vi "Select Channels Dialog.vi"(7 "Tree header":string="System Channels", 8 "error in (no error)":errorcluster, 9 "Custom Filter":refnum<k24>, 10 "Filter":u8(ring)=1 items=["K_CHAN_R", "K_CHAN_W", "K_CHAN_RW", "K_CHAN_VOLT", "K_CHAN_FAULT", "K_ALL", "K_CUSTOM"], 11 "Start Item Ref":T1=18446744073709551615 format="%.0x") -> (0 "error out":errorcluster, 1 "Canceled":bool, 3 "Channel paths":string[](array[string]))   [LabVIEW 2026, in "Nominal Core Streaming System Explorer.lvlib"]
uses:
  <vilib>/NI VeriStand/Custom Device API/Custom Device Item Ref.ctl
  NationalInstruments.VeriStand.SystemStorage
  Nominal Core Streaming System Explorer.lvlib
  <vilib>/NI VeriStand/Custom Device API/Custom Device API.lvlib
  NationalInstruments.VeriStand.SystemStorageUI
panel:
  in  "OK":bool
  in  "Cancel":bool
  in  "System Channels":refnum<k24>(container)
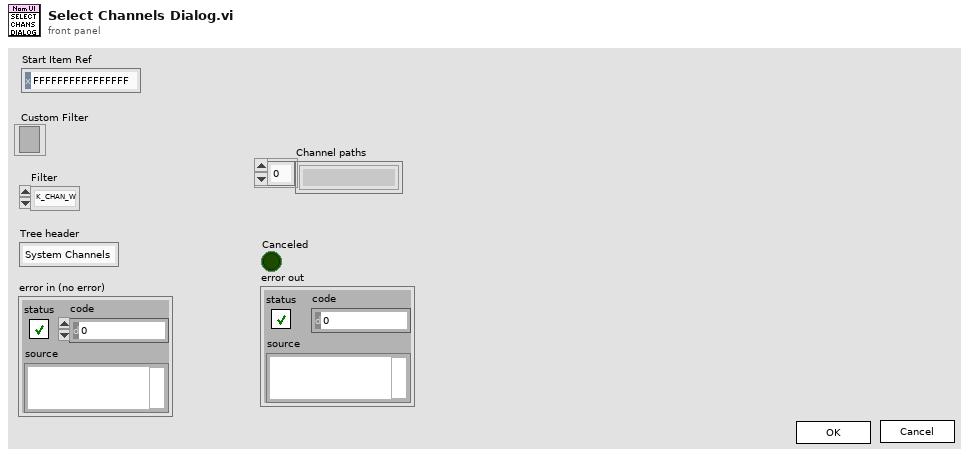
[diagram p1: front panel]
types:
  T1 = typedef "Custom Device API.lvlib/Custom Device Item Ref.ctl" = u64
  T2 = cluster{"Shut Down":bool, "Error":errorcluster, "Root":refnum<k24>, "Cancel":bool, "MapTree":cluster{"Ref":refnum<k24>, "Filter":refnum<k24>}, "Channels":string[]}
  T3 = typedef "Custom Device API.lvlib/Custom Device Pointer.ctl" = refnum<k24>
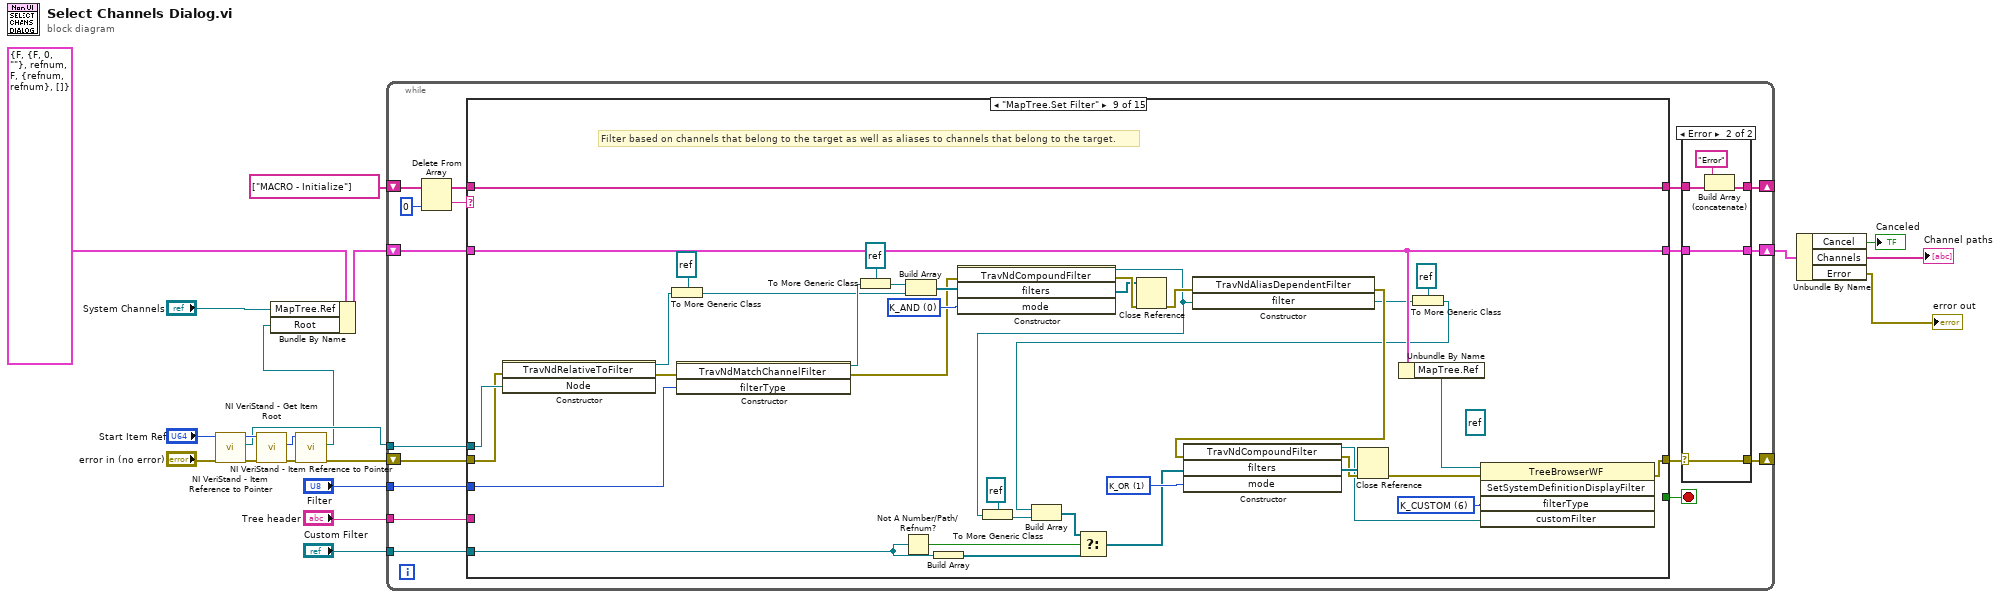
[diagram p0: block diagram]
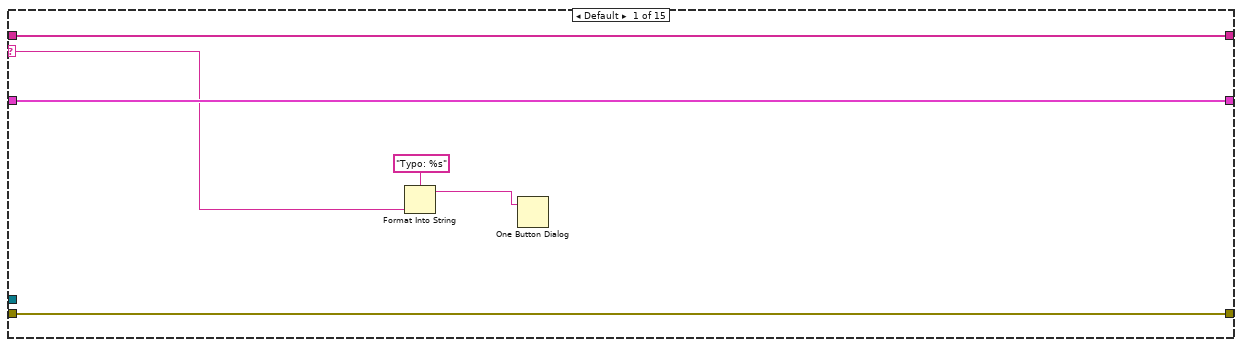
[diagram p3: hidden frame]
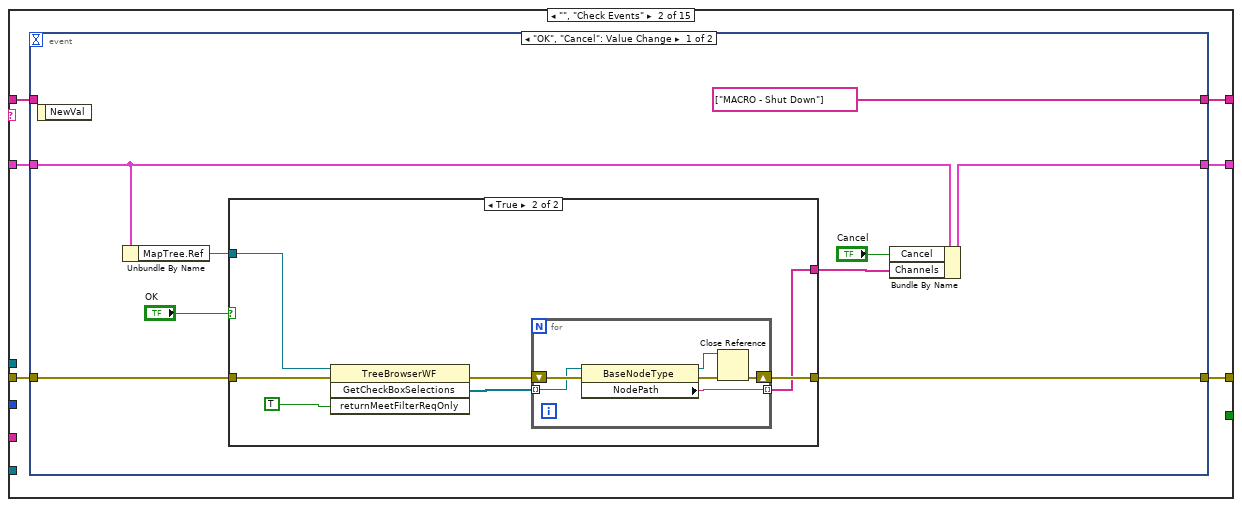
[diagram p4: hidden frame]
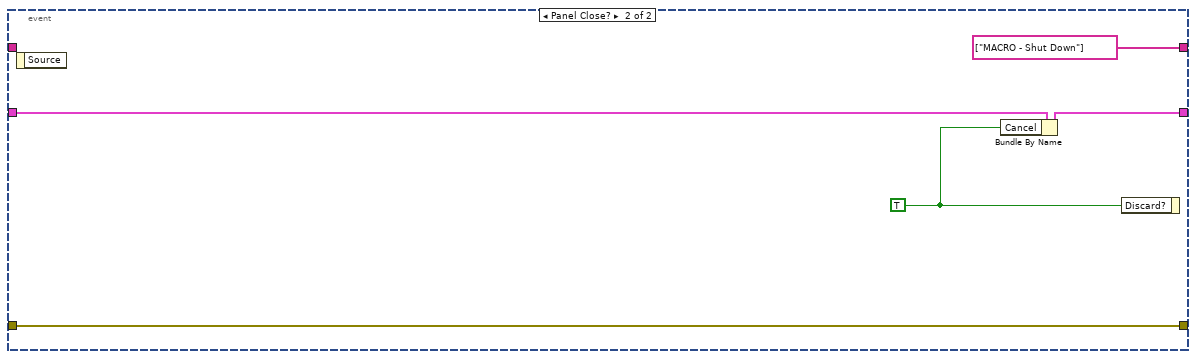
[diagram p6: hidden frame]
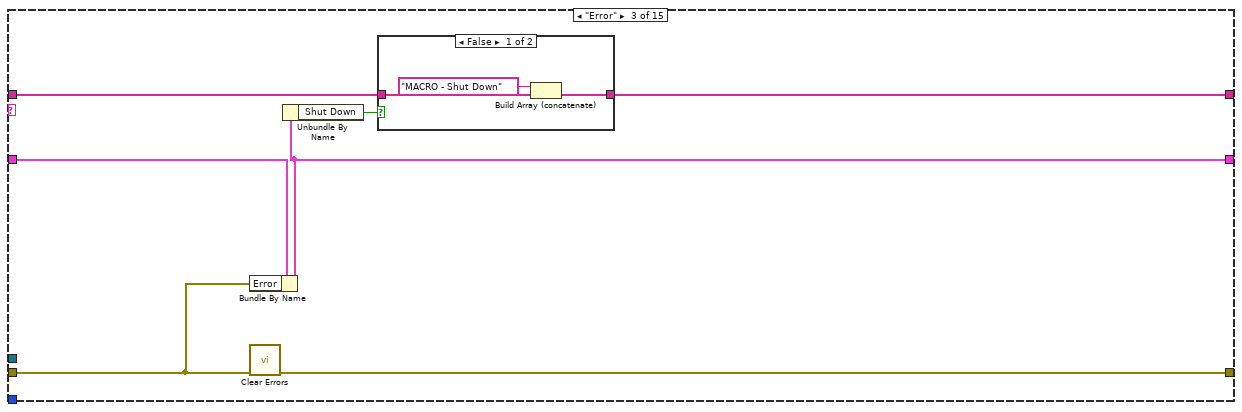
[diagram p7: hidden frame]
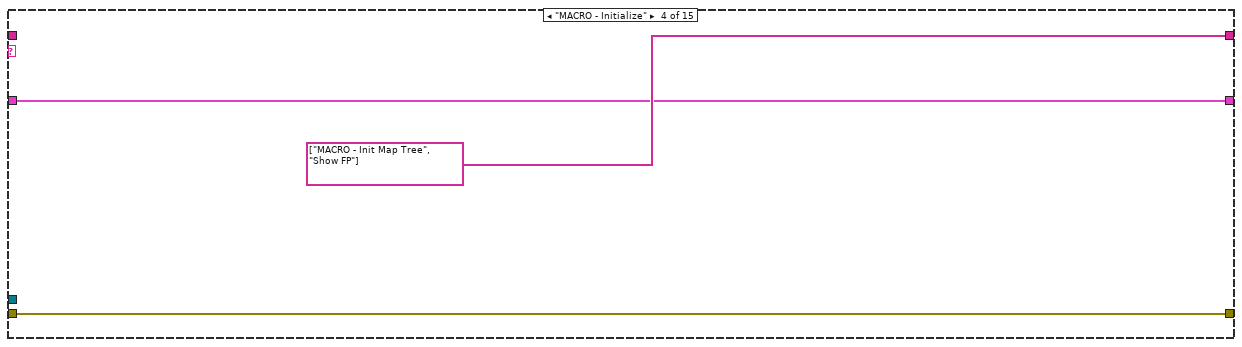
[diagram p9: hidden frame]
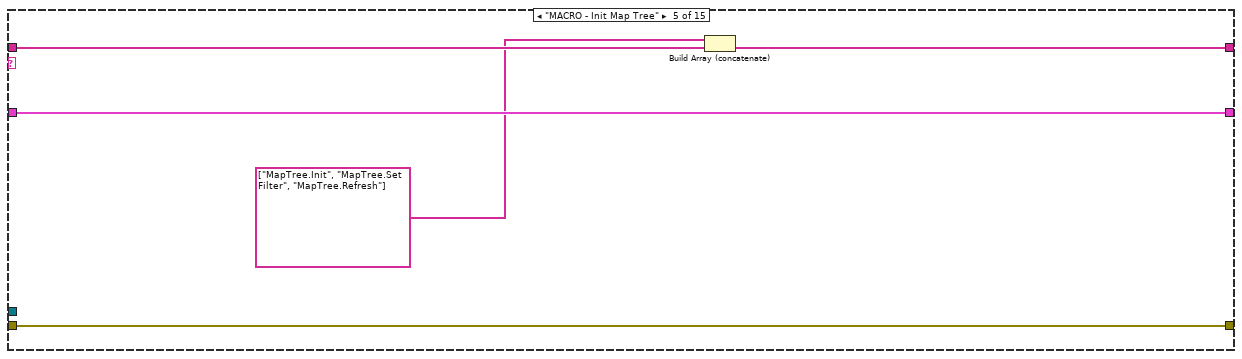
[diagram p10: hidden frame]
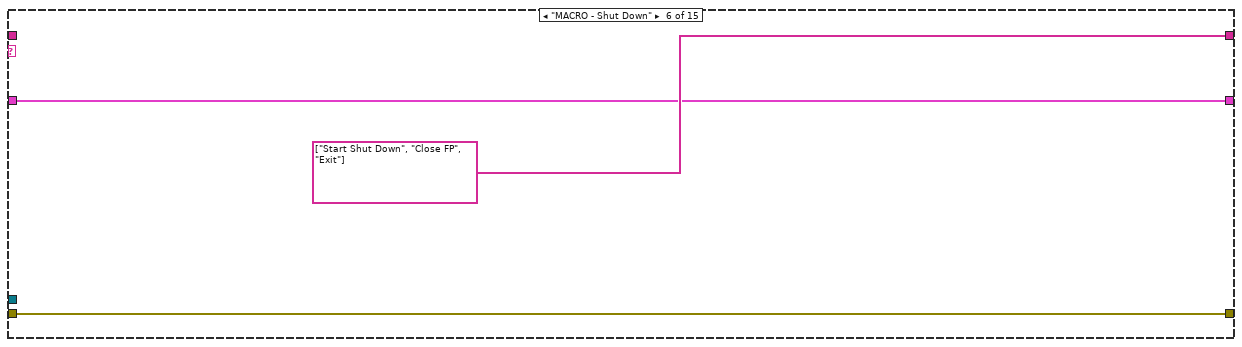
[diagram p11: hidden frame]
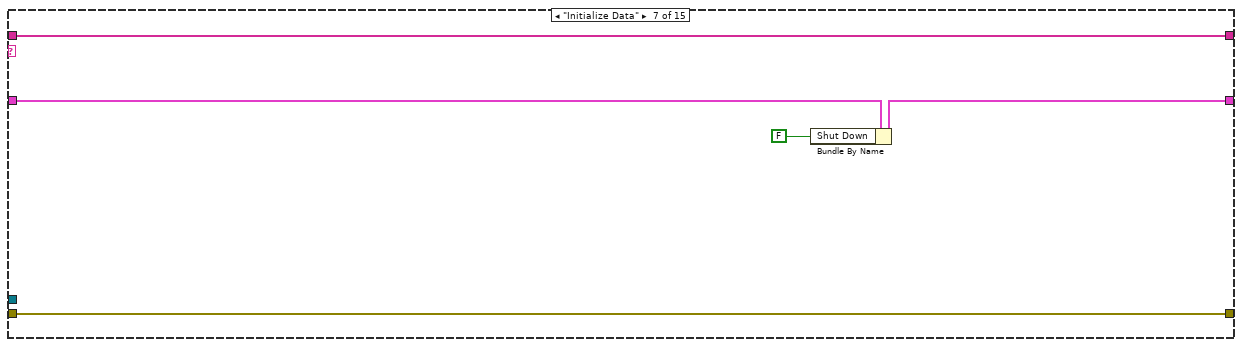
[diagram p12: hidden frame]
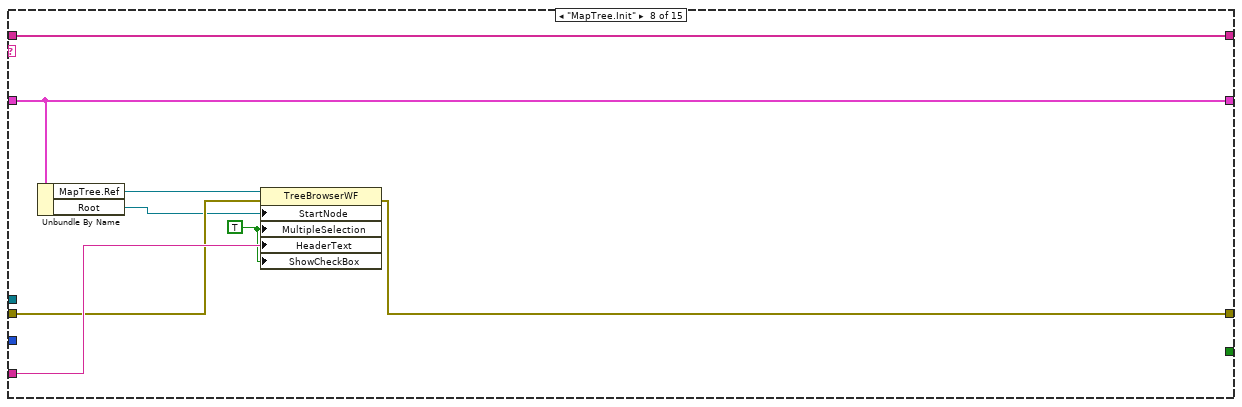
[diagram p13: hidden frame]
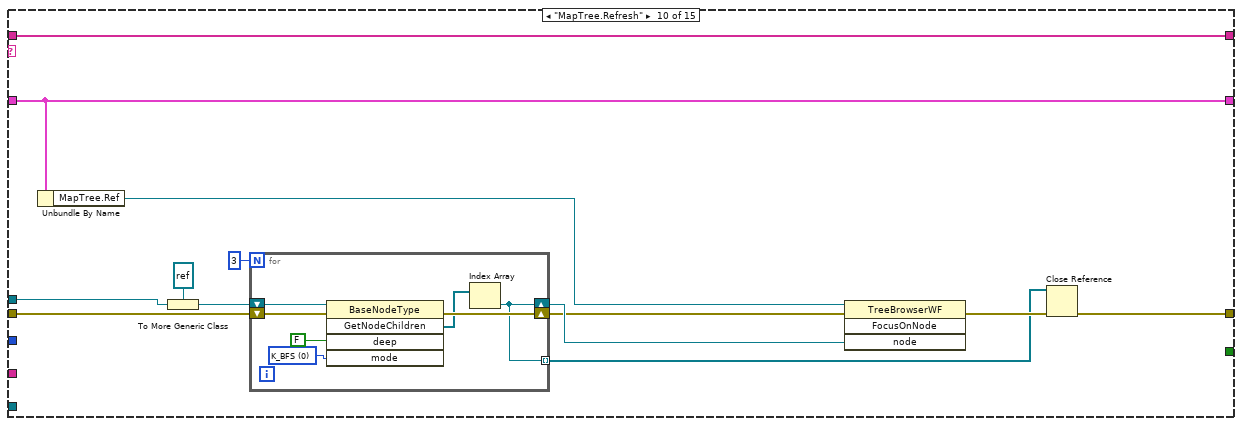
[diagram p14: hidden frame]
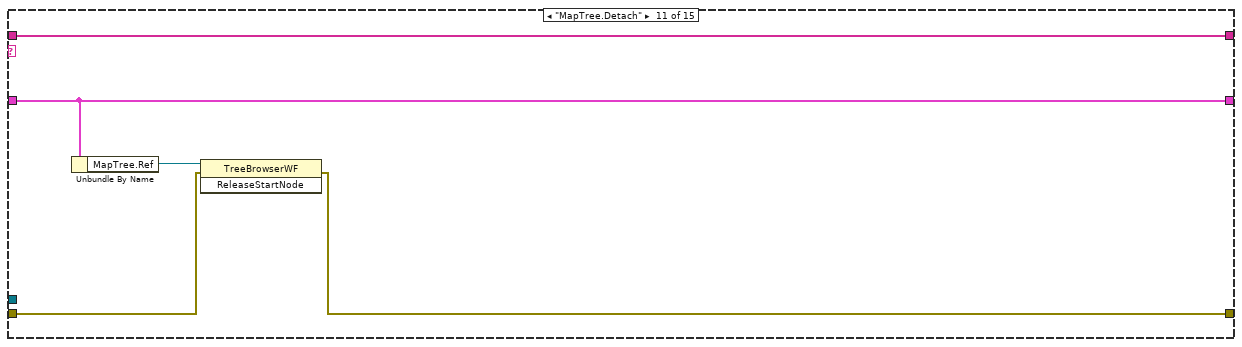
[diagram p15: hidden frame]
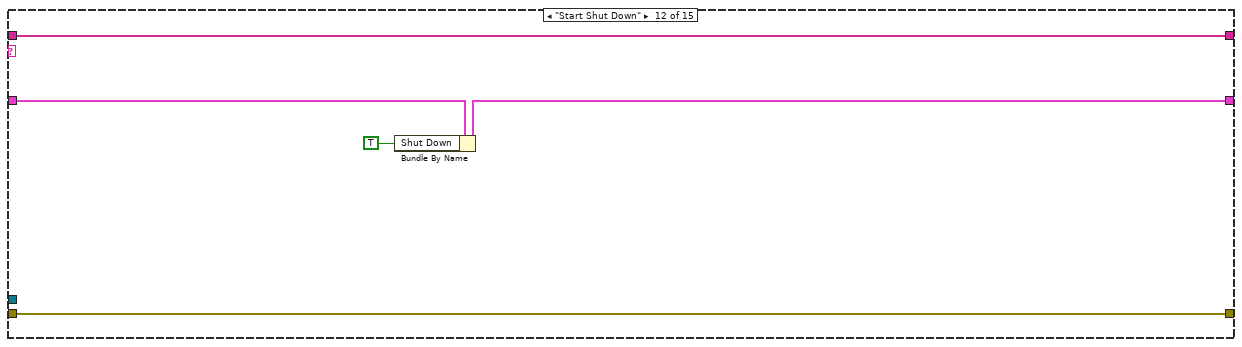
[diagram p16: hidden frame]
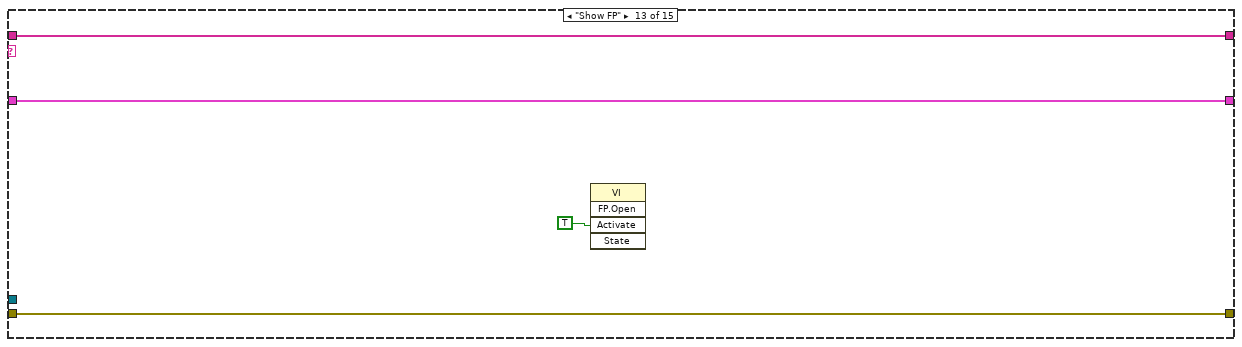
[diagram p17: hidden frame]
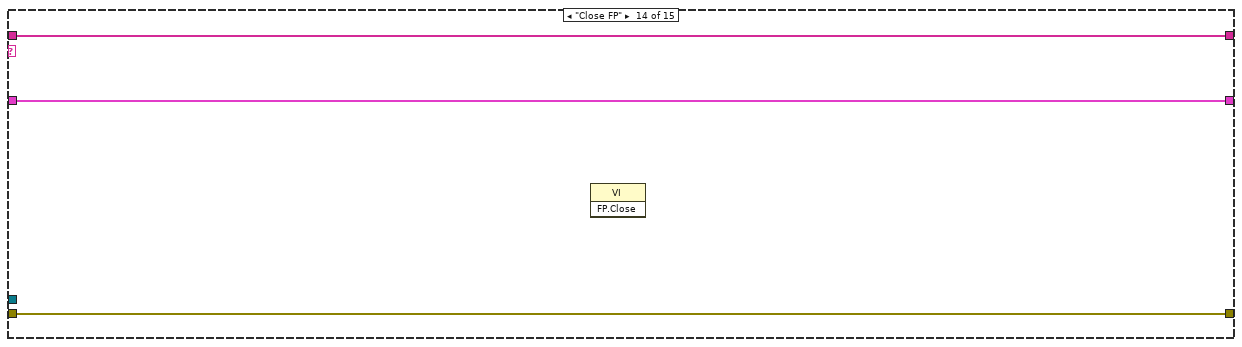
[diagram p18: hidden frame]
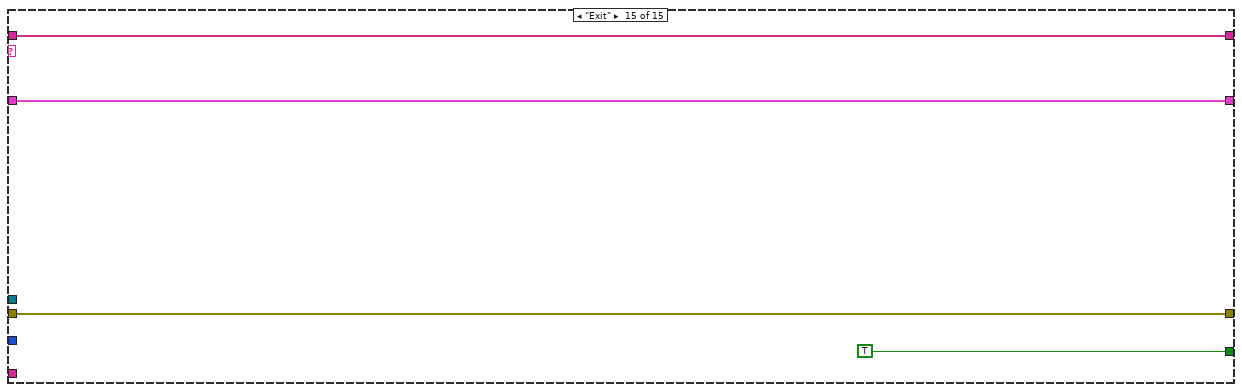
[diagram p19: hidden frame]
diagram:
  n1 = call <vilib>:"NI VeriStand - Item Reference to Pointer.vi"("error in (no error)"="error in (no error)", "Item Ref in"="Start Item Ref") -> ("error out"=w7:errorcluster, "Node Pointer"=w5:T3, "Item Ref out"=w8:T1)  [unwired: 6 in, 1 out]
  n2 = call <vilib>:"NI VeriStand - Get Item Root.vi"("error in (no error)"=w7, "Item Ref in"=w8) -> ("error out"=w4:errorcluster, "Root Ref out"=w1:T1)  [unwired: 6 in, 2 out]
  n3 = call <vilib>:"NI VeriStand - Item Reference to Pointer.vi"("error in (no error)"=w4, "Item Ref in"=w1) -> ("error out"=w3:errorcluster, "Node Pointer"=w2:T3)  [unwired: 6 in, 2 out]
  n4 = Bundle By Name(cluster=T2 {"Shut Down"=FALSE, "Error"={"status"=FALSE, "code"=0, "source"=""}, "Root"=refnum, "Cancel"=FALSE, "MapTree"={"Ref"=refnum, "Filter"=refnum}, "Channels"=[]} ("State Data"), "MapTree.Ref"="System Channels", "Root"=w2) -> (w17:T2)
  n5 = while {
    shift-right: [w27] -> _
    shift-left: string[] ["MACRO - Initialize"] -> [w37]
    shift-right: [w29] -> _
    shift-left: w3 -> [w33]
    shift-right: [w26] -> w13
    shift-left: w17 -> [w31]
    tunnel: "Tree header" -> [w24]
    tunnel: "Filter" -> [w23]
    tunnel: "Custom Filter" -> [w22]
    tunnel: w5 -> [w21]
    stop <- w32 stop-if-true
    n6 = Delete From Array(array=w37, index=0) -> (deleted portion=w34:string, array with subset deleted=w35:string[])  [unwired: 1 in]
    n7 = case shown="\"MapTree.Set Filter\"" w34 {
      selector: w34 -> [w47 _ _ _ _ _ _ _ _ _ _ _ _ _ _]
      tunnel: w35 -> [w51 w57 w89 _ w104 _ w112 w120 w158 w171 w183 w184 w192 w195 w199]
      tunnel: [w51 w52 w88 string[] ["MACRO - Init Map Tree", "Show FP"] ("array") w101 string[] ["Start Shut Down", "Close FP", "Exit"] ("array") w112 w120 w158 w171 w183 w184 w192 w195 w199] -> w28
      tunnel: [w50 w55 w86 w99 w103 w107 w111 w114 w157 w162 w179 w188 w191 w194 w198] -> w30
      tunnel: w33 -> [w50 w54 w87 w99 w103 w107 w111 w115 w129 w169 w180 w188 w191 w194 w198]
      tunnel: [_ _ _ _ _ _ _ _ _ _ _ _ _ _ TRUE] -> w32
      tunnel: w31 -> [w49 w56 w92 w97 w102 w105 w108 w119 w156 w170 w182 w187 w190 w193 w196]
      tunnel: [w49 w53 w91 w97 w102 w105 w110 w119 w156 w170 w182 w186 w190 w193 w196] -> w25
      tunnel: w24 -> [_ _ _ _ _ _ _ w117 _ _ _ _ _ _ _]
      tunnel: w23 -> [_ _ _ _ _ _ _ _ w149 _ _ _ _ _ _]
      tunnel: w22 -> [_ _ _ _ _ _ _ _ w133 _ _ _ _ _ _]
      tunnel: w21 -> [_ _ _ _ _ _ _ _ w145 w159 _ _ _ _ _]
      frame Default {
        n8 = Format Into String(format string="Typo: %s", w47) -> (resulting string=w46:string)  [unwired: 2 in, 1 out]
        n9 = One Button Dialog(message=w46) -> ()  [unwired: 1 in, 1 out]
      }
      frame "", "Check Events" {
        n10 = event shown="[0] \"OK\", \"Cancel\": Value Change" {
          selector: _ -> [_ _]
          dyn-events: _ -> [_ _]
          timeout: _ -> [_ _]
          tunnel: [w59 w85] -> w55
          tunnel: w54 -> [w61 w85]
          tunnel: [w65 w82] -> w53
          tunnel: w56 -> [w63 w84]
          tunnel: w57 -> [_ _]
          tunnel: [string[] ["MACRO - Shut Down"] string[] ["MACRO - Shut Down"]] -> w52
          event "OK", "Cancel": Value Change {
            n11 = event-data() -> ()  [unwired: 1 in, 1 out]
            n12 = Unbundle By Name(w63) -> ("MapTree.Ref"=w62:refnum<k24>)
            n13 = case shown="True" "OK" {
              tunnel: w62 -> [_ w74]
              tunnel: w61 -> [w67 w73]
              tunnel: [_ w68] -> w60
              tunnel: [w67 w69] -> w59
              frame False {
              }
              frame True {
                n14 = invoke class="TreeBrowserWF" method="GetCheckBoxSelections"(reference=w74, error in=w73, "returnMeetFilterReqOnly"=TRUE) -> (error out=w71:errorcluster, "GetCheckBoxSelections"=w70:refnum<k24>[])  [unwired: 1 in, 2 out]
                n15 = for {
                  shift-right: [w75] -> w69
                  shift-left: w71 -> [w80]
                  tunnel: w70 -> [w79] mode=indexing
                  tunnel: [w78] -> w68 mode=indexing
                  n16 = property class="BaseNodeType"(reference=w79, error in=w80) -> (reference out=w76:refnum<k24>, error out=w77:errorcluster, "NodePath"=w78:string)
                  n17 = Close Reference(reference=w76, error in (no error)=w77) -> (error out=w75:errorcluster)
                }
              }
            }
            n18 = Bundle By Name(cluster=w63, "Cancel"="Cancel", "Channels"=w60) -> (w65:T2)
          }
          event Panel Close? {
            w81 = TRUE ("Discard?")
            n19 = event-data() -> ()  [unwired: 1 in, 1 out]
            n20 = Bundle By Name(cluster=w84, "Cancel"=w81) -> (w82:T2)
            n21 = event-data("Discard?"=w81) -> ()  [unwired: 1 in, 1 out]
          }
        }
      }
      frame "Error" {
        n22 = Bundle By Name(cluster=w92, "Error"=w87) -> (w91:T2)
        n23 = call <vilib>:"Clear Errors.vi"("error in (no error)"=w87) -> ("error out"=w86:errorcluster)  [unwired: 5 in, 1 out]
        n24 = Unbundle By Name(w91) -> ("Shut Down"=w90:bool)
        n25 = case shown="False" w90 {
          tunnel: w89 -> [w94 w96]
          tunnel: [w93 w96] -> w88
          frame False {
            n26 = Build Array (concatenate)("MACRO - Shut Down", w94) -> (w93:string[])
          }
          frame True {
            # "Do not interrupt a shut down sequence. This can cause an infinite loop."
          }
        }
      }
      frame "MACRO - Initialize" {
      }
      frame "MACRO - Init Map Tree" {
        n27 = Build Array (concatenate)(string[] ["MapTree.Init", "MapTree.Set Filter", "MapTree.Refresh"] ("array"), w104) -> (w101:string[])
      }
      frame "MACRO - Shut Down" {
      }
      frame "Initialize Data" {
        n28 = Bundle By Name(cluster=w108, "Shut Down"=FALSE) -> (w110:T2)
      }
      frame "MapTree.Init" {
        w116 = TRUE ("MultipleSelection")
        n29 = Unbundle By Name(w119) -> ("MapTree.Ref"=w118:refnum<k24>, "Root"=w113:refnum<k24>)
        n30 = property class="TreeBrowserWF"(reference=w118, error in=w115, "StartNode"=w113, "MultipleSelection"=w116, "HeaderText"=w117, "ShowCheckBox"=w116) -> (error out=w114:errorcluster)  [unwired: 1 out]
      }
      frame "MapTree.Set Filter" {
        (unwired) refnum<k24> refnum ("MapTree.Ref")
        w146 = 0 items=["K_AND", "K_OR"] ("mode")
        w148 = u8 6 items=["K_CHAN_R", "K_CHAN_W", "K_CHAN_RW", "K_CHAN_VOLT", "K_CHAN_FAULT", "K_ALL", "K_CUSTOM", "K_CHAN_R_VIS", "K_CHAN_W_VIS", "K_CHAN_RW_VIS", "K_CHAN_VOLT_VIS", "K_CHAN_FAULT_VIS", "K_WAVE", "K_WAVE_VIS", "K_WAVE_DBL", "K_WAVE_CDB", "K_WAVE_DBL_VIS", "K_WAVE_CDB_VIS"] ("filterType")
        w153 = 1 items=["K_AND", "K_OR"] ("mode")
        # "Filter based on channels that belong to the target as well as aliases to channels that belong to the target."
        n31 = constructor class="TravNdRelativeToFilter"(error in=w129, "Node"=w145) -> (reference out=w142:refnum<k24>, error out=w128:errorcluster)  [unwired: 2 in, 2 out]
        n32 = To More Generic Class(target class=refnum<k24> refnum ("new reference"), reference=w142) -> (generic class reference=w130:refnum<k24>)
        n33 = constructor class="TravNdMatchChannelFilter"(error in=w128, "filterType"=w149) -> (reference out=w144:refnum<k24>, error out=w127:errorcluster)  [unwired: 2 in, 2 out]
        n34 = To More Generic Class(target class=refnum<k24> refnum ("new reference"), reference=w144) -> (generic class reference=w131:refnum<k24>)
        n35 = Not A Number/Path/Refnum?(number/path/refnum=w133) -> (NaN/Path/Refnum?=w134:bool)
        n36 = Build Array(w131, w130) -> (w141:refnum<k24>[])
        n37 = Build Array(w133) -> (w122:refnum<k24>[])
        n38 = constructor class="TravNdCompoundFilter"(error in=w127, "filters"=w141, "mode"=w146) -> (reference out=w123:refnum<k24>, error out=w140:errorcluster, "filters"=w139:refnum<k24>[])  [unwired: 2 in, 2 out]
        n39 = To More Generic Class(target class=refnum<k24> refnum ("new reference"), reference=w123) -> (generic class reference=w124:refnum<k24>)
        n40 = Close Reference(reference=w139, error in (no error)=w140) -> (error out=w138:errorcluster)
        n41 = constructor class="TravNdAliasDependentFilter"(error in=w138, "filter"=w123) -> (reference out=w136:refnum<k24>, error out=w155:errorcluster)  [unwired: 2 in, 2 out]
        n42 = Unbundle By Name(w156) -> ("MapTree.Ref"=w147:refnum<k24>)
        n43 = To More Generic Class(target class=refnum<k24> refnum ("new reference"), reference=w136) -> (generic class reference=w126:refnum<k24>)
        n44 = Build Array(w126, w124) -> (w121:refnum<k24>[])
        n45 = Select(t=w121, s=w134, f=w122) -> (s? t:f=w132:refnum<k24>[])
        n46 = constructor class="TravNdCompoundFilter"(error in=w155, "filters"=w132, "mode"=w153) -> (reference out=w135:refnum<k24>, error out=w151:errorcluster, "filters"=w152:refnum<k24>[])  [unwired: 2 in, 2 out]
        n47 = Close Reference(reference=w152, error in (no error)=w151) -> (error out=w150:errorcluster)
        n48 = invoke class="TreeBrowserWF" method="SetSystemDefinitionDisplayFilter"(reference=w147, error in=w150, "filterType"=w148, "customFilter"=w135) -> (error out=w157:errorcluster)  [unwired: 1 in, 4 out]
      }
      frame "MapTree.Refresh" {
        n49 = Unbundle By Name(w170) -> ("MapTree.Ref"=w160:refnum<k24>)
        n50 = To More Generic Class(target class=refnum<k24> refnum, reference=w159) -> (generic class reference=w167:refnum<k24>)
        n51 = for {
          N: 3 -> [_]
          shift-right: [w172] -> w166
          shift-left: w167 -> [w175]
          shift-right: [w178] -> w161
          shift-left: w169 -> [w174]
          tunnel: [w172] -> w163 mode=indexing
          w176 = 0 items=["K_BFS", "K_DFS", "K_CHILDONLY", "K_UP"] ("mode")
          n52 = invoke class="BaseNodeType" method="GetNodeChildren"(reference=w175, error in=w174, "deep"=FALSE, "mode"=w176) -> (error out=w178:errorcluster, "GetNodeChildren"=w173:refnum<k24>[])  [unwired: 1 in, 3 out]
          n53 = Index Array(array=w173) -> (element=w172:refnum<k24>)  [unwired: 1 in]
        }
        n54 = invoke class="TreeBrowserWF" method="FocusOnNode"(reference=w160, error in=w161, "node"=w166) -> (error out=w164:errorcluster)  [unwired: 1 in, 3 out]
        n55 = Close Reference(reference=w163, error in (no error)=w164) -> (error out=w162:errorcluster)
      }
      frame "MapTree.Detach" {
        n56 = Unbundle By Name(w182) -> ("MapTree.Ref"=w181:refnum<k24>)
        n57 = invoke class="TreeBrowserWF" method="ReleaseStartNode"(reference=w181, error in=w180) -> (error out=w179:errorcluster)  [unwired: 1 in, 2 out]
      }
      frame "Start Shut Down" {
        n58 = Bundle By Name(cluster=w187, "Shut Down"=TRUE) -> (w186:T2)
      }
      frame "Show FP" {
        n59 = invoke class="VI" method="FP.Open"("Activate"=TRUE ("Activate?")) -> ()  [unwired: 4 in, 5 out]
      }
      frame "Close FP" {
        n60 = invoke class="VI" method="FP.Close"() -> ()  [unwired: 3 in, 3 out]
      }
      frame "Exit" {
      }
    }
    n61 = case shown="Error" w30 {
      selector: w30 -> [w40 w45]
      tunnel: [w40 w45] -> w29
      tunnel: w28 -> [w39 w43]
      tunnel: [w39 w42] -> w27
      tunnel: [w38 w44] -> w26
      tunnel: w25 -> [w38 w44]
      frame No Error {
      }
      frame Error {
        n62 = Build Array (concatenate)("Error", w43) -> (w42:string[])
      }
    }
  }
  n63 = Unbundle By Name(w13) -> ("Cancel"=→"Canceled":bool, "Channels"=→"Channel paths":string[], "Error"=→"error out":errorcluster)
